vi "OAT Compensate Even Angle Signal (Vector Ref, N Channels).vi"(0 "even-angle signals":cluster{"r0":dbl, "dr":dbl, "Y":dbl[]}[](array[cluster]) {"r0" format="%.2p"; "dr" format="%.2p"; "Y" format="%.2f"}, 1 "orders to compensate":dbl[](array[numeric]) format="%.2f", 2 "reset? (F)":bool, 5 "vector references":cdb[][](array[numeric]) format="%.2f", 7 "even-angle position info":T1, 9 "speed profile":T2 {"speed [RPM]" format="%.2f"; "time [s]" format="%.2f"}, 11 "error in (no error)":errorcluster) -> (4 "compensated even-angle signals":cluster{"r0":dbl, "dr":dbl, "Y":dbl[]}[](array[cluster]) {"r0" format="%.2p"; "dr" format="%.2p"; "Y" format="%.2f"}, 6 "actual vector references":cdb[][](array[numeric]) format="%.2f", 8 "even-angle position info out":T1, 15 "error out":errorcluster)   [LabVIEW 2017, in "SoundVib_RefDataProcess.lvlib"]
doc: "Compensates an even-angle signal. You can use the <B>compensated even-angle signal</B> output to display unfiltered orbit and timebase plots with the runout pattern removed. Wire data to the <B>even-angle signal</B> input to determine the polymorphic instance to use or manually select the instance."
uses:
  <vilib>/addons/Sound and Vibration/Order Analysis/Referece Data Processing/SoundVib_RefDataProcess.lvlib
  <vilib>/addons/Sound and Vibration/Order Analysis/Misc/OAT Position Info.ctl
  <vilib>/addons/Sound and Vibration/Order Analysis/Tach Process/SubVIs/speed profile.ctl
  <vilib>/addons/Sound and Vibration/Order Analysis/Resample Order Tracking/SoundVib_Resampling.lvlib
  <vilib>/addons/Sound and Vibration/Order Analysis/Tach Process/SoundVib_TachProcess.lvlib
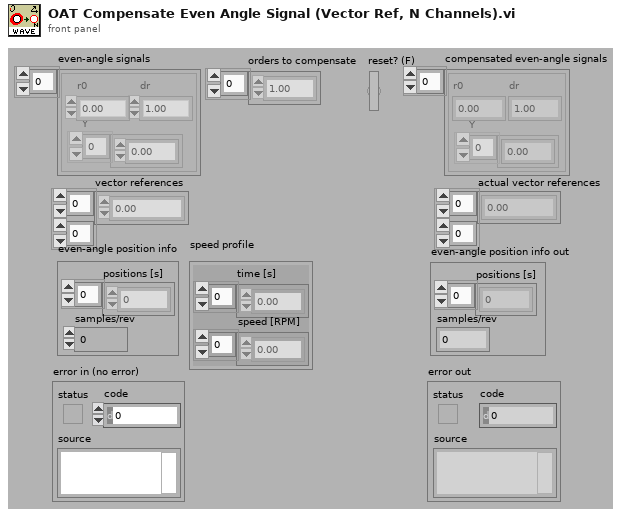
[diagram p1: front panel]
types:
  T1 = typedef "OAT Position Info.ctl" = cluster{"positions [s]":dbl[], "samples/rev":dbl}
  T2 = typedef "SoundVib_TachProcess.lvlib/speed profile.ctl" = cluster{"time [s]":dbl[], "speed [RPM]":dbl[]}
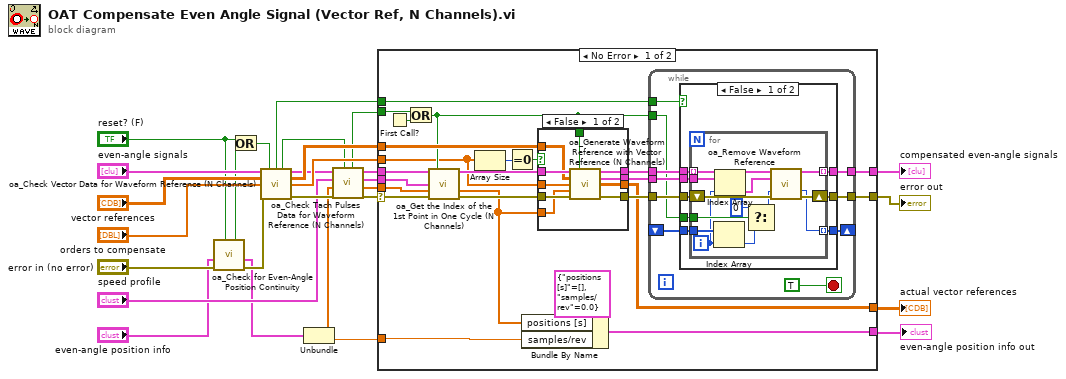
[diagram p0: block diagram]
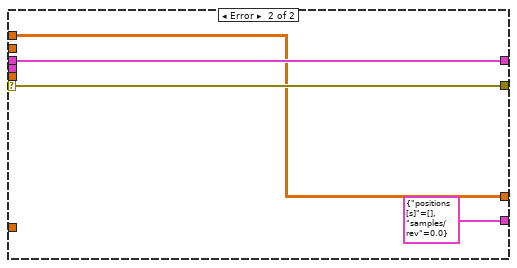
[diagram p4: hidden frame]
diagram:
  n1 = call <vilib>:"oa_Check for Even-Angle Position Continuity.vi"("reset in"="reset? (F)", "error in (no error)"="error in (no error)", "even-angle position info"="even-angle position info") -> ("error out"=w6:errorcluster, "even-angle position info dup"=w4:T1, "position not continuous"=w2:bool)  [unwired: 6 in]
  n2 = Or(x="reset? (F)", y=w2) -> (x .or. y?=w1:bool)
  n3 = call <vilib>:"oa_Check Vector Data for Waveform Reference (N Channels).vi"("resampled signal"="even-angle signals", "reset? (True)"=w1, "slow roll vectors"="vector references", "orders to compensate"="orders to compensate", "error out in"=w6) -> ("empty signal?"=w10:bool, "parameter changed"=w16:bool, "resampled signal dup"=w20:cluster{"r0":dbl, "dr":dbl, "Y":dbl[]}[], "slow roll vectors dup"=w25:cdb[][], "orders to compensate dup"=w24:dbl[], "error out"=w18:errorcluster)  [unwired: 5 in]
  n4 = Unbundle(w4) -> ("positions [s]"=w12:dbl[], "samples/rev"=w9:dbl)
  n5 = call <vilib>:"oa_Check Tach Pulses Data for Waveform Reference (N Channels).vi"("reset? (True)"=w16, "error in (no error)"=w18, "interpolated pulse positions"=w12, "speed profile"="speed profile", "even angle signals"=w20) -> ("error out"=w17:errorcluster, "interpolated pulse positions out"=w11:dbl[], "speed profile out"=w13:T2, "even angle signals"=w19:cluster{"r0":dbl, "dr":dbl, "Y":dbl[]}[], "reset"=w15:bool)  [unwired: 2 in]
  n6 = case shown="No Error" w17 {
    selector: w17 -> [w51 w102]
    tunnel: w19 -> [w52 w103]
    tunnel: w25 -> [w41 w101]
    tunnel: w24 -> [w37 _]
    tunnel: w13 -> [w43 _]
    tunnel: w11 -> [w33 _]
    tunnel: [w35 w101] -> w23
    tunnel: [w50 w103] -> w22
    tunnel: [w49 w102] -> w21
    tunnel: w15 -> [w38 _]
    tunnel: w10 -> [w34 _]
    tunnel: w9 -> [w30 _]
    tunnel: [w29 T1 {"positions [s]"=[], "samples/rev"=0.0} ("even angle position info")] -> w8
    frame No Error {
      n7 = First Call?() -> (First Call?: T/F=w39:bool)
      n8 = Or(x=w38, y=w39) -> (x .or. y?=w40:bool)
      n9 = call <vilib>:"oa_Get the Index of the 1st Point in One Cycle (N Channels).vi"("resampled signal"=w52, "reset? (True)"=w40, "speed profile"=w43, "interpolated pulse positions"=w33, "error in (no error)"=w51) -> ("resampled signal out"=w48:cluster{"r0":dbl, "dr":dbl, "Y":dbl[]}[], "interpolated pulse positions out"=w31:dbl[], "error out"=w47:errorcluster)  [unwired: 8 in]
      n10 = Array Size(array=w37) -> (size(s)=w36:i32)
      n11 = Equal To 0?(x=w36) -> (x = 0?=w42:bool)
      n12 = Bundle By Name(cluster=T1 {"positions [s]"=[], "samples/rev"=0.0} ("even angle position info"), "positions [s]"=w31, "samples/rev"=w30) -> (w29:T1)
      n13 = case shown="False" w42 {
        tunnel: w48 -> [w62 w65]
        tunnel: w40 -> [w61 _]
        tunnel: [w60 w65] -> w46
        tunnel: w47 -> [w59 w64]
        tunnel: [w58 w64] -> w44
        tunnel: [w57 _] -> w45
        tunnel: w37 -> [w56 _]
        tunnel: w31 -> [w53 _]
        tunnel: w41 -> [w55 w63]
        tunnel: [w54 w63] -> w35
        frame False {
          n14 = call <vilib>:"oa_Generate Waveform Reference with Vector Reference (N Channels).vi"("resampled signal"=w62, "reset? (True)"=w61, "slow roll vectors"=w55, "orders to compensate"=w56, "interpolated positions [s]"=w53, "error out in"=w59) -> ("resampled signal out"=w60:cluster{"r0":dbl, "dr":dbl, "Y":dbl[]}[], "reference signal out"=w57:cluster{"r0":dbl, "dr":dbl, "Y":dbl[]}[], "slow roll vectors out"=w54:cdb[][], "error out"=w58:errorcluster)  [unwired: 6 in]
        }
        frame True {
        }
      }
      n15 = while {
        shift-right: [w70] -> _
        shift-left: _ -> [w68]
        tunnel: w40 -> [w67]
        tunnel: w44 -> [w73]
        tunnel: [w72] -> w49
        tunnel: w45 -> [w69]
        tunnel: w34 -> [w66]
        tunnel: w46 -> [w75]
        tunnel: [w71] -> w50
        stop <- TRUE stop-if-true
        n16 = case shown="False" w66 {
          tunnel: w75 -> [w83 w99]
          tunnel: w73 -> [w82 w98]
          tunnel: [w81 w98] -> w72
          tunnel: [w80 w99] -> w71
          tunnel: [w79 w97] -> w70
          tunnel: w69 -> [w78 _]
          tunnel: w68 -> [w77 w97]
          tunnel: w67 -> [w76 _]
          frame False {
            n17 = for {
              tunnel: w83 -> [w96] mode=indexing
              tunnel: [w93] -> w80 mode=indexing
              shift-right: [w94] -> w81
              shift-left: w82 -> [w95]
              tunnel: [w92] -> w79 mode=indexing
              tunnel: w78 -> [w86]
              tunnel: w77 -> [w88]
              tunnel: w76 -> [w90]
              i -> [w85]
              n18 = Index Array(array=w88, index=w85) -> (element=w87:i32)
              n19 = Index Array(array=w86, index=w85) -> (element=w84:cluster{"r0":dbl, "dr":dbl, "Y":dbl[]})
              n20 = Select(t=0, s=w90, f=w87) -> (s? t:f=w89:i32)
              n21 = call <vilib>:"oa_Remove Waveform Reference.vi"("resampled signal"=w96, "baseline in"=w84, "last index"=w89, "error out in"=w95) -> ("compensated signal"=w93:cluster{"r0":dbl, "dr":dbl, "Y":dbl[]}, "last index out"=w92:i32, "error out"=w94:errorcluster)  [unwired: 9 in]
            }
          }
          frame True {
          }
        }
      }
    }
    frame Error {
    }
  }
  "error out" <- w21
  "compensated even-angle signals" <- w22
  "actual vector references" <- w23
  "even-angle position info out" <- w8
